vi "TwoProtocolLoop.vi"() -> ()   [LabVIEW 2018]
panel:
  out "current repeat":dbl
  in  "num repeats":dbl
  in  "protocol2 name":string
  in  "protocol1 name":string
  in  "delay after protocol2 (ms)":dbl
  in  "delay after protocol1 (ms)":dbl
  in  "initial delay (ms)":dbl
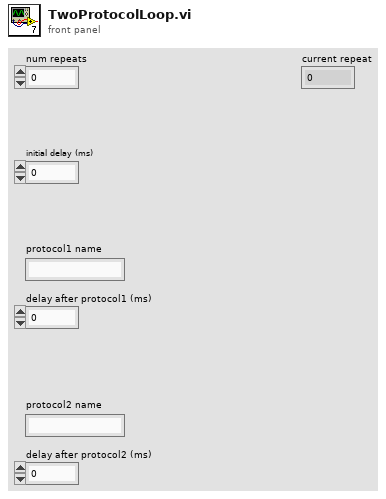
[diagram p1: front panel]
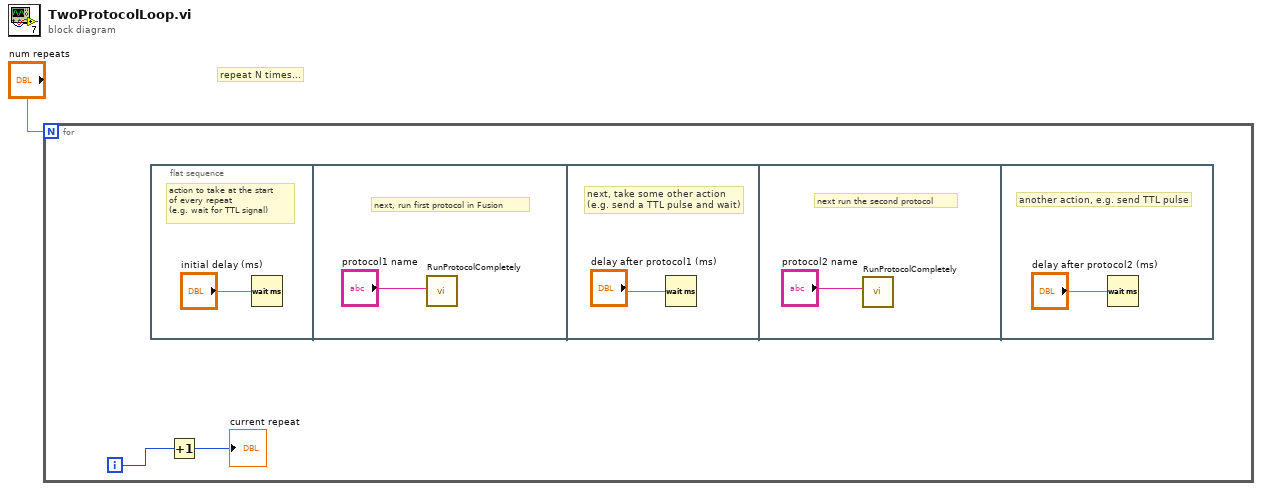
[diagram p0: block diagram]
diagram:
  # "repeat N times..."
  n1 = for {
    N: "num repeats" -> [_]
    i -> [w3]
    n2 = flat-sequence {
      frame #0 {
        # "action to take at the start\nof every repeat\n(e.g. wait for TTL signal)"
        n3 = Wait (ms)(milliseconds to wait="initial delay (ms)") -> ()  [unwired: 1 out]
      }
      frame #1 {
        # "next, run first protocol in Fusion"
        n4 = call "RunProtocolCompletely.vi"("protocol name"="protocol1 name") -> ()  [unwired: 11 in]
      }
      frame #2 {
        # "next, take some other action\n(e.g. send a TTL pulse and wait)"
        n5 = Wait (ms)(milliseconds to wait="delay after protocol1 (ms)") -> ()  [unwired: 1 out]
      }
      frame #3 {
        # "next run the second protocol"
        n6 = call "RunProtocolCompletely.vi"("protocol name"="protocol2 name") -> ()  [unwired: 11 in]
      }
      frame #4 {
        # "another action, e.g. send TTL pulse"
        n7 = Wait (ms)(milliseconds to wait="delay after protocol2 (ms)") -> ()  [unwired: 1 out]
      }
    }
    n8 = Increment(x=w3) -> (x+1=→"current repeat":i32)
  }
